vi "Auto Probe Sense Value.vi"(8 "error in (no error)":errorcluster {"code" format="%.0x"}, 10 "Channel (\"Channel 1\")":string(combo)="CHAN1", 11 "VISA Resource Name":refnum<visa-resource-name>) -> (0 "error out":errorcluster {"code" format="%.0x"}, 2 "auto probe sense value":dbl caption="Auto Probe Sense Value" format="%^.2e", 3 "VISA Resource Name Out":refnum<visa-resource-name>)   [LabVIEW 2011, in "Agilent 546XX Series.lvlib"]
doc: "The VI returns the probe attenuation value the oscilloscope senses."
uses:
  Agilent 546XX Series.lvlib
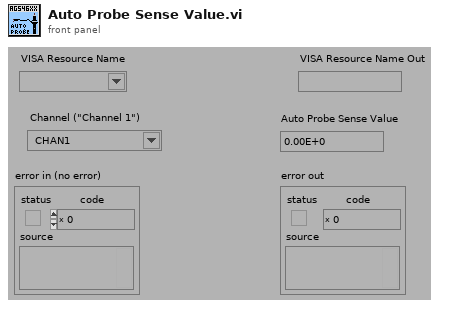
[diagram p1: front panel]
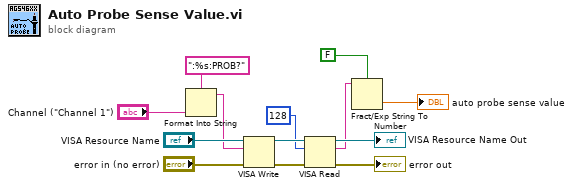
[diagram p0: block diagram]
diagram:
  n1 = Format Into String(format string=":%s:PROB?", "Channel (\"Channel 1\")") -> (resulting string=w5:string)  [unwired: 2 in, 1 out]
  n2 = VISA Write(VISA resource name="VISA Resource Name", write buffer=w5, error in (no error)="error in (no error)") -> (VISA resource name out=w13:refnum<visa-resource-name>, error out=w12:errorcluster)  [unwired: 1 out]
  n3 = VISA Read(VISA resource name=w13, byte count=u32 128, error in (no error)=w12) -> (VISA resource name out=→"VISA Resource Name Out":refnum<visa-resource-name>, read buffer=w3:string, error out=→"error out":errorcluster)  [unwired: 1 out]
  n4 = Fract/Exp String To Number(use system decimal point (T)=FALSE, string=w3) -> (number=→"auto probe sense value":dbl)  [unwired: 2 in, 1 out]
